vi "LoadControlValues.vi"(7 "Axis":T1=1 items=["Axis Control"=0, "Axis 1"=1, "Axis 2"=2, "Axis 3"=3, "Axis 4"=4, "Axis 5"=5, "Axis 6"=6, "Axis 7"=7, "Axis 8"=8, "Vector Space Control"=16, "Vector Space 1"=17, "Vector Space 2"=18, "Vector Space 3"=19, "Vector Space 4"=20, "Encoder Control"=32, "Encoder 1"=33, "Encoder 2"=34, "Encoder 3"=35, "Encoder 4"=36, "Encoder 5"=37, "Encoder 6"=38, "Encoder 7"=39, "Encoder 8"=40, "DAC Channel 1"=49, "DAC Channel 2"=50, "DAC Channel 3"=51, "DAC Channel 4"=52, "DAC Channel 5"=53, "DAC Channel 6"=54, "DAC Channel 7"=55, "DAC Channel 8"=56, "Stepper Output 1"=65, "Stepper Output 2"=66, "Stepper Output 3"=67, "Stepper Output 4"=68, "Stepper Output 5"=69, "Stepper Output 6"=70, "Stepper Output 7"=71, "Stepper Output 8"=72, "ADC Channel 1"=81, "ADC Channel 2"=82, "ADC Channel 3"=83, "ADC Channel 4"=84, "ADC Channel 5"=85, "ADC Channel 6"=86, "ADC Channel 7"=87, "ADC Channel 8"=88], 8 "error in (no error)":errorcluster, 11 "path":path) -> (0 "error out":errorcluster)   [LabVIEW 2010]
uses:
  <vilib>/Motion/FlexMotion/CustomControls/CustomControls.llb/Resource Out (Enum).flx
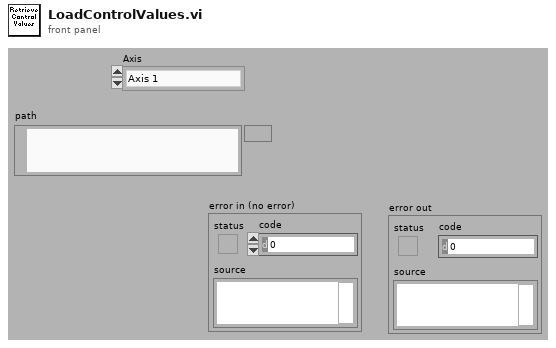
[diagram p1: front panel]
types:
  T1 = typedef "Resource Out (Enum).flx" = u16
  T2 = cluster{"Name":string, "type string":i16[], "data string":string}[]
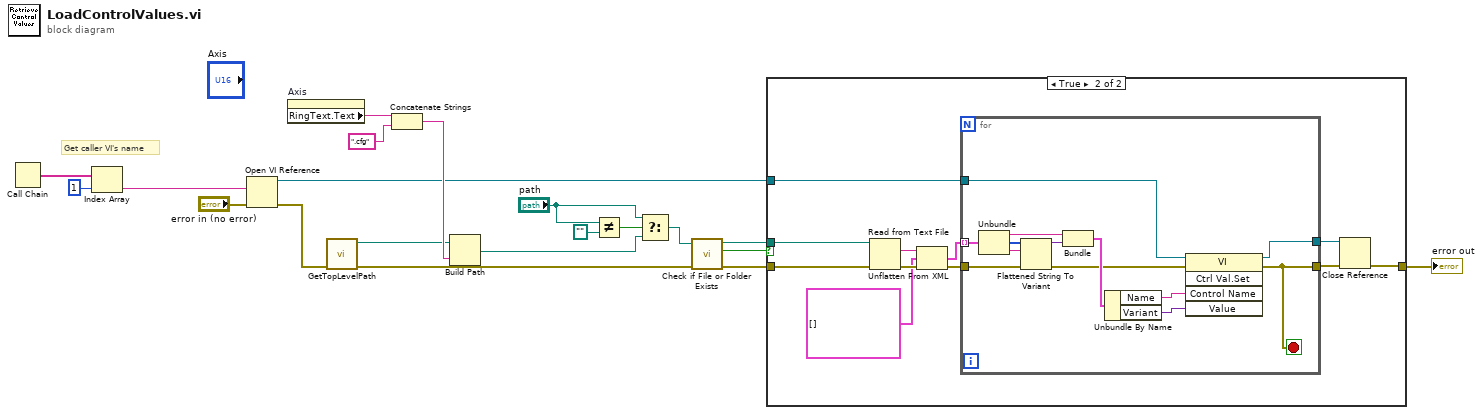
[diagram p0: block diagram]
diagram:
  # "Get caller VI's name"
  n1 = Call Chain() -> (call chain=w8:string[])
  n2 = Index Array(array=w8, index=1) -> (element=w6:string)
  n3 = Open VI Reference(vi path=w6, error in (no error)="error in (no error)") -> (vi reference=w5:refnum<vi>, error out=w4:errorcluster)  [unwired: 4 in]
  n4 = property on="Axis" class="Ring (strict)"() -> ("RingText.Text"=w1:string)  [unwired: 2 in, 2 out]
  n5 = call "GetTopLevelPath.vi"("error in"=w4) -> ("error out"=w3:errorcluster, "path"=w2:path)  [unwired: 9 in]
  n6 = Concatenate Strings(w1, ".cfg" ("string")) -> (w14:string)
  n7 = Build Path(base path=w2, name or relative path=w14) -> (appended path=w10:path)
  n8 = Not Equal?(x="path", y=path "") -> (x != y?=w13:bool)
  n9 = Select(t="path", s=w13, f=w10) -> (s? t:f=w9:path)
  n10 = call <vilib>:"Check if File or Folder Exists.vi"("error in (no error)"=w3, "path"=w9) -> ("error out"=w16:errorcluster, "file or folder exists?"=w18:bool, "dup path"=w19:path)  [unwired: 7 in]
  n11 = case shown="True" w18 {
    tunnel: w5 -> [_ w27]
    tunnel: w19 -> [_ w26]
    tunnel: w16 -> [w21 w25]
    tunnel: [w21 w24] -> w7
    frame False {
    }
    frame True {
      n12 = Read from Text File(file (use dialog)=w26, error in=w25) -> (text=w32:string, error out=w30:errorcluster)  [unwired: 4 out]
      n13 = Unflatten From XML(xml string=w32, type=T2 [], error in (no error)=w30) -> (value=w28:T2, error out=w31:errorcluster)
      n14 = for {
        tunnel: w31 -> [w44]
        tunnel: [w33] -> w23
        tunnel: w28 -> [w41] mode=indexing
        tunnel: w27 -> [w35]
        tunnel: [w34] -> w22
        stop <- w33 stop-if-true
        n15 = Unbundle(w41) -> ("Name"=w42:string, "type string"=w40:i16[], "data string"=w39:string)
        n16 = Flattened String To Variant(4:w44, 6:w39, 7:w40) -> (0:w36:errorcluster, 3:w43:variant)
        n17 = Bundle("Name"=w42, "Variant"=w43) -> (w38:cluster{"Name":string, "Variant":variant})  [unwired: 1 out]
        n18 = Unbundle By Name(w38) -> ("Name"=w37:string, "Variant"=w45:variant)
        n19 = invoke class="VI" method="Ctrl Val.Set"(reference=w35, error in=w36, "Control Name"=w37, "Value"=w45) -> (reference out=w34:refnum<vi>, error out=w33:errorcluster)  [unwired: 1 in, 3 out]
      }
      n20 = Close Reference(reference=w22, error in (no error)=w23) -> (error out=w24:errorcluster)
    }
  }
  "error out" <- w7
